vi "test Action Update Heater State-Enable Heater.vi"() -> ()   [LabVIEW 2018, in "Action Update Heater State.lvclass"]
uses:
  Action Update Heater State.lvclass
  Libraries/Thermal Chamber Controller_DQMH/Heater State--enum.ctl
  Libraries/Thermal Chamber Controller_DQMH/Thermal Chamber Controller_DQMH.lvlib
  Libraries/Thermal Chamber Response Simulator/Thermal Chamber Response Simulator.lvlib
panel:
  out "TestCase out":refnum<class "Action Update Heater State.lvclass">
  in  "TestCase in":refnum<class "Action Update Heater State.lvclass">
  out "error out":errorcluster
  in  "error in (no error)":errorcluster
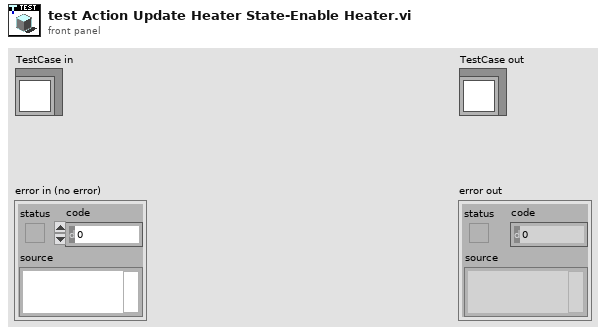
[diagram p1: front panel]
types:
  T1 = typedef "Thermal Chamber Controller_DQMH.lvlib/Heater State--enum.ctl" = enum16{"Heater Enabled", "Heater Disabled"}
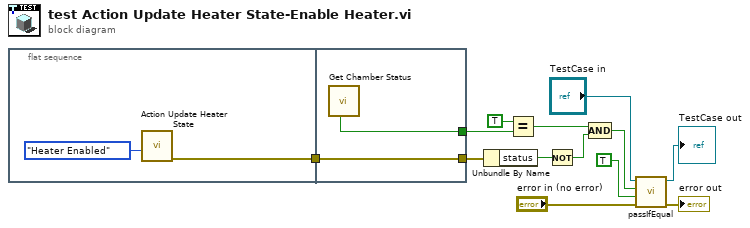
[diagram p0: block diagram]
diagram:
  n1 = flat-sequence {
    tunnel: [w14] -> w4
    tunnel: [w17] -> w7
    tunnel: w4 -> [w17]
    tunnel: [w16] -> w3
    frame #0 {
      n2 = call "Action Update Heater State.vi"("Heater State"=Heater_State--enum."Heater Enabled" ("Heater State Result")) -> ("error out"=w14:errorcluster)  [unwired: 10 in]
    }
    frame #1 {
      n3 = call "Get Chamber Status.vi"() -> ("Heater State"=w16:bool)  [unwired: 6 in, 5 out]
    }
  }
  n4 = Unbundle By Name(w7) -> ("status"=w10:bool)
  n5 = Equal?(x=TRUE, y=w3) -> (x = y?=w9:bool)
  n6 = Not(x=w10) -> (.not. x?=w6:bool)
  n7 = Compound Arithmetic op=AND(w9, w6) -> (w5:bool)
  n8 = call-dynamic "passIfEqual.vi"("error in (no error)"="error in (no error)", "y"=TRUE, "x"=w5, "TestCase in"="TestCase in") -> ("error out"=→"error out":errorcluster, "TestCase out"=→"TestCase out":refnum<class "Action Update Heater State.lvclass">)  [unwired: 6 in]
